vi "Clear Output.vi"(0 "PainOutputTerminal in":refnum<class "SystemLinkOutputTerminal.lvclass">, 11 "error in (no error)":errorcluster) -> (4 "PainOutputTerminal out":refnum<class "SystemLinkOutputTerminal.lvclass">, 15 "error out":errorcluster)   [LabVIEW 2016, in "SystemLinkOutputTerminal.lvclass"]
uses:
  SystemLinkOutputTerminal.lvclass
  Plain OT/PainOutputTerminal.lvclass
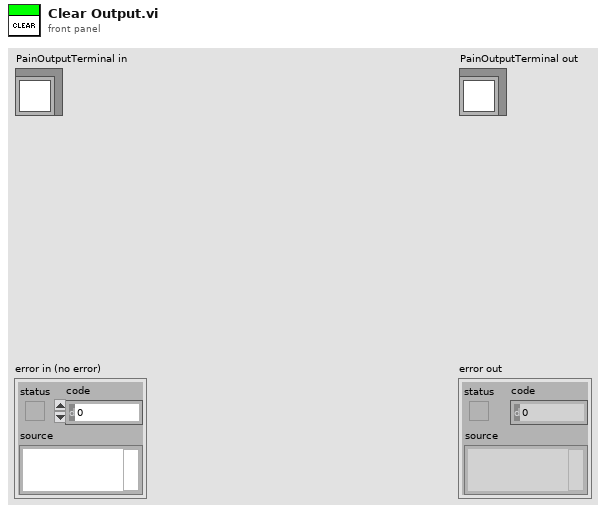
[diagram p1: front panel]
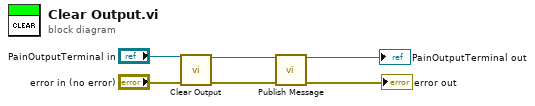
[diagram p0: block diagram]
diagram:
  n1 = call-parent "Clear Output.vi"("PainOutputTerminal in"="PainOutputTerminal in", "error in (no error)"="error in (no error)") -> ("PainOutputTerminal out"=w4:refnum<class "SystemLinkOutputTerminal.lvclass">, "error out"=w1:errorcluster)  [unwired: 12 in]
  n2 = call "Publish Message.vi"("SystemLinkOutputTerminal in"=w4, "error in (no error)"=w1) -> ("SystemLinkOutputTerminal out"=→"PainOutputTerminal out":refnum<class "SystemLinkOutputTerminal.lvclass">, "error out"=→"error out":errorcluster)  [unwired: 12 in]
